vi "Action Name.vi"(8 "error in (no error)":errorcluster, 11 "Filter by Is Receive In":refnum<class "Filter by Is Receive.lvclass">) -> (0 "error out":errorcluster, 2 "Action Name":string, 3 "Filter by Is Receive Out":refnum<class "Filter by Is Receive.lvclass">)   [LabVIEW 2020, in "Filter by Is Receive.lvclass"]
uses:
  Filter by Is Receive.lvclass
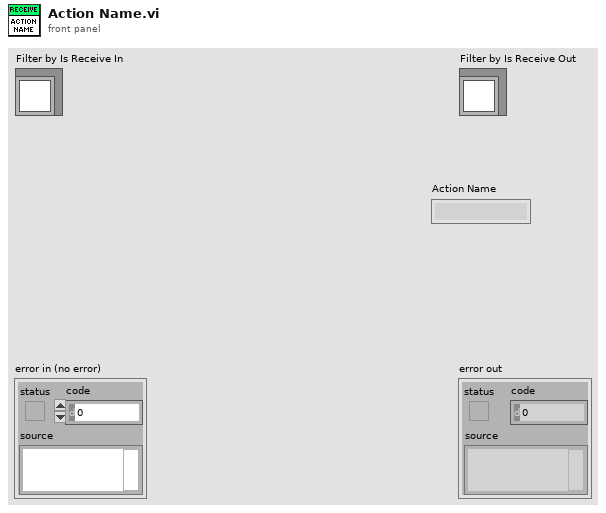
[diagram p1: front panel]
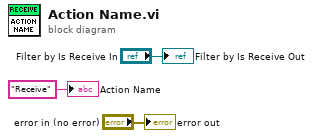
[diagram p0: block diagram]
diagram:
  "error out" <- "error in (no error)"
  "Filter by Is Receive Out" <- "Filter by Is Receive In"
  "Action Name" <- "Receive"
